vi "subGoRef.vi"(1 "AxisId":i32=1 min=1 max=6, 2 "Index":i32=1) -> ()   [LabVIEW 2020]
panel:
  in  "ref8":bool caption="search for min. reference switch, search for max. reference switch, then set counter to zero"
  in  "ref7":bool caption="search for max. reference switch, search for min. reference switch, then set counter to zero"
  in  "ref6":bool caption="search for reference switch and next index impulse (as type 3), then set counter to zero"
  in  "ref5":bool caption="search for reference switch (as type 2) and set counter to zero"
  in  "ref4":bool caption="search for next index impulse (as type 1) and set counter to zero"
  in  "ref3":bool caption="search for reference switch and next index impulse, then stop"
  in  "ref2":bool caption="search for reference switch and release"
  in  "ref1":bool caption="search for next index impulse and stop"
  in  "Start":bool
  in  "Close":bool
  # "Type of the reference run"
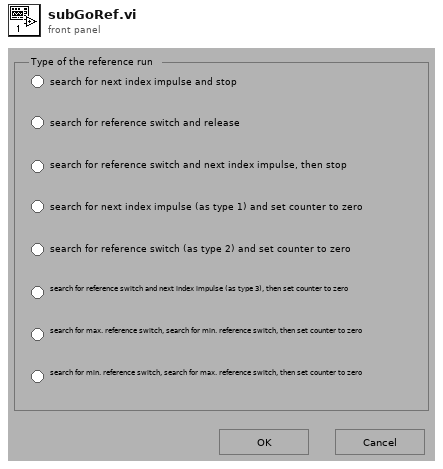
[diagram p1: front panel]
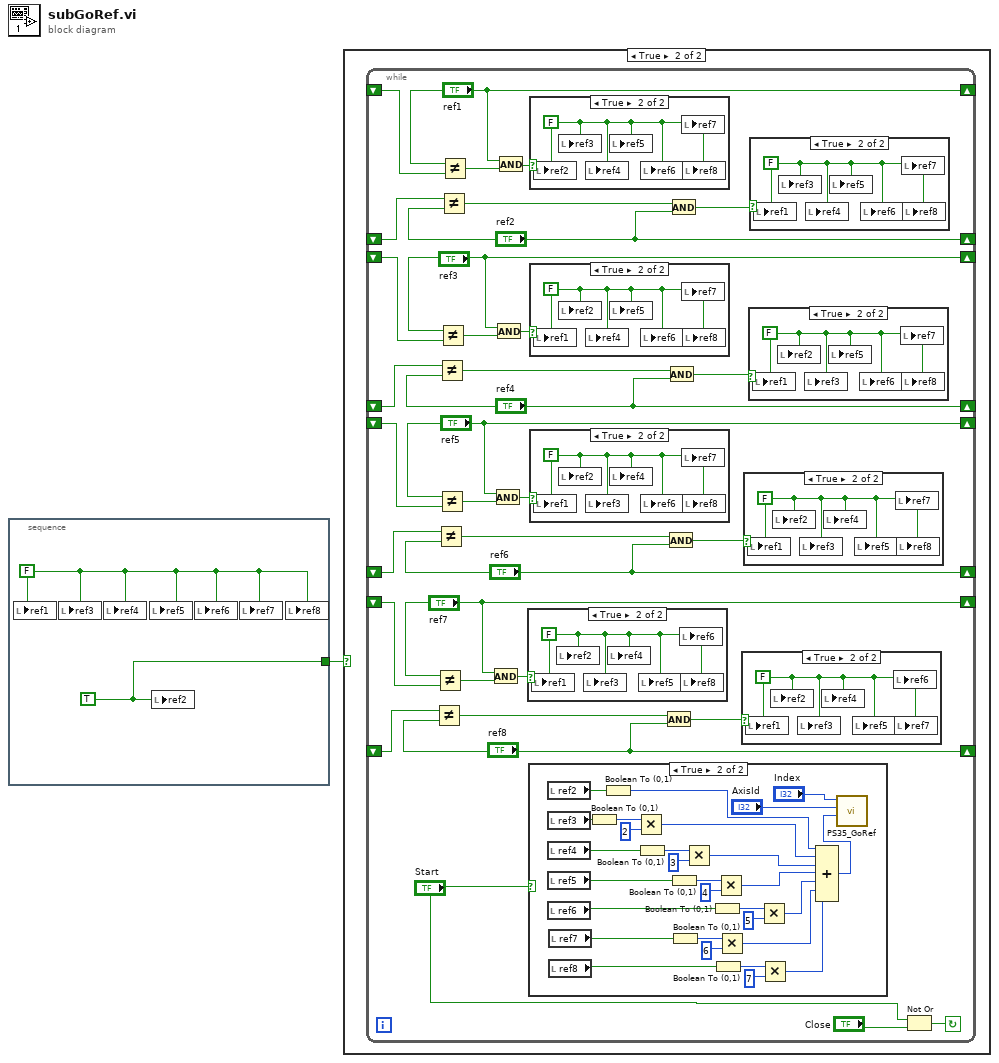
[diagram p0: block diagram]
diagram:
  n1 = stacked-sequence {
    tunnel: [w3] -> w1
    frame #0 {
      w3 = TRUE ("WriteRead")
      w2 = FALSE ("WriteRead")
      n2 = local write "ref1"(w2) -> ()
      n3 = local write "ref3"(w2) -> ()
      n4 = local write "ref4"(w2) -> ()
      n5 = local write "ref5"(w2) -> ()
      n6 = local write "ref2"(w3) -> ()
      n7 = local write "ref6"(w2) -> ()
      n8 = local write "ref7"(w2) -> ()
      n9 = local write "ref8"(w2) -> ()
    }
  }
  n10 = case shown="True" w1 {
    frame False {
    }
    frame True {
      n11 = while {
        shift-left: _ -> [w9]
        shift-right: ["ref7"] -> _
        shift-left: _ -> [w7]
        shift-right: ["ref8"] -> _
        shift-left: _ -> [w20]
        shift-right: ["ref1"] -> _
        shift-left: _ -> [w22]
        shift-right: ["ref2"] -> _
        shift-left: _ -> [w29]
        shift-right: ["ref3"] -> _
        shift-left: _ -> [w27]
        shift-right: ["ref4"] -> _
        shift-left: _ -> [w31]
        shift-right: ["ref5"] -> _
        shift-left: _ -> [w33]
        shift-right: ["ref6"] -> _
        stop <- w38 continue-if-true
        n12 = Not Equal?(x=w7, y="ref8") -> (x != y?=w6:bool)
        n13 = Not Equal?(x="ref7", y=w9) -> (x != y?=w8:bool)
        n14 = Not Equal?(x=w33, y="ref6") -> (x != y?=w35:bool)
        n15 = Not Equal?(x=w27, y="ref4") -> (x != y?=w26:bool)
        n16 = Not Equal?(x="ref5", y=w31) -> (x != y?=w32:bool)
        n17 = Not Equal?(x="ref3", y=w29) -> (x != y?=w28:bool)
        n18 = Not Equal?(x=w22, y="ref2") -> (x != y?=w23:bool)
        n19 = Not Equal?(x="ref1", y=w20) -> (x != y?=w21:bool)
        n20 = And(x="ref7", y=w8) -> (x .and. y?=w10:bool)
        n21 = And(x="ref5", y=w32) -> (x .and. y?=w13:bool)
        n22 = And(x="ref3", y=w28) -> (x .and. y?=w15:bool)
        n23 = And(x="ref1", y=w21) -> (x .and. y?=w17:bool)
        n24 = case shown="True" w10 {
          frame False {
          }
          frame True {
            w39 = FALSE ("WriteRead")
            n25 = local write "ref1"(w39) -> ()
            n26 = local write "ref2"(w39) -> ()
            n27 = local write "ref3"(w39) -> ()
            n28 = local write "ref4"(w39) -> ()
            n29 = local write "ref5"(w39) -> ()
            n30 = local write "ref6"(w39) -> ()
            n31 = local write "ref8"(w39) -> ()
          }
        }
        n32 = case shown="True" "Start" {
          frame False {
          }
          frame True {
            n33 = local read "ref2"() -> (w72:bool)
            n34 = local read "ref3"() -> (w69:bool)
            n35 = local read "ref4"() -> (w62:bool)
            n36 = local read "ref5"() -> (w61:bool)
            n37 = local read "ref6"() -> (w60:bool)
            n38 = local read "ref7"() -> (w54:bool)
            n39 = local read "ref8"() -> (w55:bool)
            n40 = Boolean To (0,1)(Boolean=w69) -> (0, 1=w74:i16)
            n41 = Boolean To (0,1)(Boolean=w72) -> (0, 1=w71:i16)
            n42 = Multiply(x=w74, y=2) -> (x*y=w70:i32)
            n43 = Boolean To (0,1)(Boolean=w62) -> (0, 1=w67:i16)
            n44 = Boolean To (0,1)(Boolean=w61) -> (0, 1=w66:i16)
            n45 = Boolean To (0,1)(Boolean=w54) -> (0, 1=w50:i16)
            n46 = Multiply(x=w67, y=3) -> (x*y=w59:i32)
            n47 = Boolean To (0,1)(Boolean=w60) -> (0, 1=w63:i16)
            n48 = Boolean To (0,1)(Boolean=w55) -> (0, 1=w53:i16)
            n49 = Multiply(x=w66, y=4) -> (x*y=w58:i32)
            n50 = Multiply(x=w50, y=6) -> (x*y=w49:i32)
            n51 = Multiply(x=w63, y=5) -> (x*y=w57:i32)
            n52 = Multiply(x=w53, y=7) -> (x*y=w48:i32)
            n53 = Compound Arithmetic op=ADD(w71, w70, w59, w58, w57, w49, w48) -> (w56:i32)
            n54 = call "PS35_GoRef.vi"("Mode"=w56, "Axis number"="AxisId", "Control unit ID"="Index") -> ()  [unwired: 4 in, 1 out]
          }
        }
        n55 = case shown="True" w17 {
          frame False {
          }
          frame True {
            w46 = FALSE ("WriteRead")
            n56 = local write "ref2"(w46) -> ()
            n57 = local write "ref3"(w46) -> ()
            n58 = local write "ref4"(w46) -> ()
            n59 = local write "ref5"(w46) -> ()
            n60 = local write "ref6"(w46) -> ()
            n61 = local write "ref7"(w46) -> ()
            n62 = local write "ref8"(w46) -> ()
          }
        }
        n63 = case shown="True" w15 {
          frame False {
          }
          frame True {
            w44 = FALSE ("WriteRead")
            n64 = local write "ref1"(w44) -> ()
            n65 = local write "ref2"(w44) -> ()
            n66 = local write "ref4"(w44) -> ()
            n67 = local write "ref5"(w44) -> ()
            n68 = local write "ref6"(w44) -> ()
            n69 = local write "ref7"(w44) -> ()
            n70 = local write "ref8"(w44) -> ()
          }
        }
        n71 = case shown="True" w13 {
          frame False {
          }
          frame True {
            w42 = FALSE ("WriteRead")
            n72 = local write "ref1"(w42) -> ()
            n73 = local write "ref2"(w42) -> ()
            n74 = local write "ref3"(w42) -> ()
            n75 = local write "ref4"(w42) -> ()
            n76 = local write "ref6"(w42) -> ()
            n77 = local write "ref7"(w42) -> ()
            n78 = local write "ref8"(w42) -> ()
          }
        }
        n79 = And(x=w6, y="ref8") -> (x .and. y?=w11:bool)
        n80 = And(x=w35, y="ref6") -> (x .and. y?=w12:bool)
        n81 = And(x=w26, y="ref4") -> (x .and. y?=w14:bool)
        n82 = And(x=w23, y="ref2") -> (x .and. y?=w16:bool)
        n83 = case shown="True" w11 {
          frame False {
          }
          frame True {
            w40 = FALSE ("WriteRead")
            n84 = local write "ref1"(w40) -> ()
            n85 = local write "ref2"(w40) -> ()
            n86 = local write "ref3"(w40) -> ()
            n87 = local write "ref4"(w40) -> ()
            n88 = local write "ref5"(w40) -> ()
            n89 = local write "ref6"(w40) -> ()
            n90 = local write "ref7"(w40) -> ()
          }
        }
        n91 = case shown="True" w12 {
          frame False {
          }
          frame True {
            w41 = FALSE ("WriteRead")
            n92 = local write "ref1"(w41) -> ()
            n93 = local write "ref2"(w41) -> ()
            n94 = local write "ref3"(w41) -> ()
            n95 = local write "ref4"(w41) -> ()
            n96 = local write "ref5"(w41) -> ()
            n97 = local write "ref7"(w41) -> ()
            n98 = local write "ref8"(w41) -> ()
          }
        }
        n99 = case shown="True" w14 {
          frame False {
          }
          frame True {
            w43 = FALSE ("WriteRead")
            n100 = local write "ref1"(w43) -> ()
            n101 = local write "ref2"(w43) -> ()
            n102 = local write "ref3"(w43) -> ()
            n103 = local write "ref5"(w43) -> ()
            n104 = local write "ref6"(w43) -> ()
            n105 = local write "ref7"(w43) -> ()
            n106 = local write "ref8"(w43) -> ()
          }
        }
        n107 = case shown="True" w16 {
          frame False {
          }
          frame True {
            w45 = FALSE ("WriteRead")
            n108 = local write "ref1"(w45) -> ()
            n109 = local write "ref3"(w45) -> ()
            n110 = local write "ref4"(w45) -> ()
            n111 = local write "ref5"(w45) -> ()
            n112 = local write "ref6"(w45) -> ()
            n113 = local write "ref7"(w45) -> ()
            n114 = local write "ref8"(w45) -> ()
          }
        }
        n115 = Not Or(1:"Close", 2:"Start") -> (0:w38:bool)
      }
    }
  }
